vi "Read-Write Holding Registers.vi"(5 "write values":u16[](array[numeric]), 7 "write starting address":u16, 8 "error in (no error)":errorcluster, 9 "read quantity":u16, 10 "read starting address":u16, 11 "MB session in":refnum<class "MB_Master.lvclass">) -> (0 "error out":errorcluster, 2 "read registers":u16[](array[numeric]), 3 "MB session out":refnum<class "MB_Master.lvclass">)   [LabVIEW 2016, in "MB Master.lvlib"]
doc: "Function Code 23: Writes <b>write values</b> to holding registers starting at <b>write starting address</b> then reads <b>read quantity</b> number of holding registers starting at <b>read starting address</b>"
uses:
  MB Master.lvlib
  MB_Master.lvclass
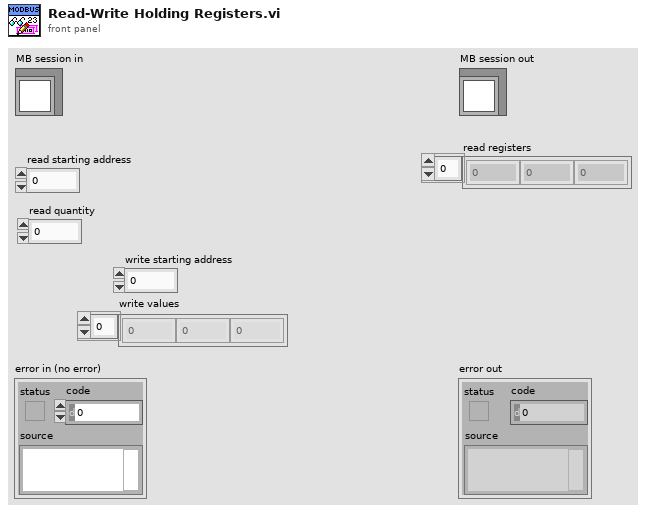
[diagram p1: front panel]
types:
  T1 = typedef "MB Master.lvlib/MB_PDU_Cluster.ctl" = cluster{"Function Code":u8, "Data":u8[], "RTU_DataBytes":i32}
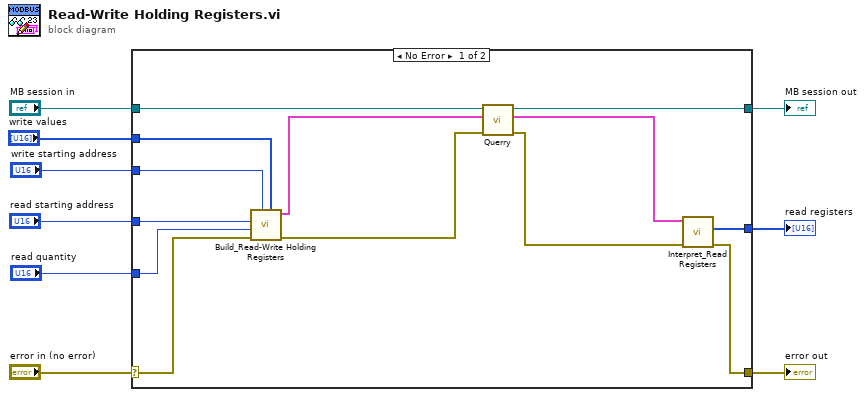
[diagram p0: block diagram]
diagram:
  n1 = case shown="No Error" "error in (no error)" {
    selector: "error in (no error)" -> [w14 w24]
    tunnel: [w21 w24] -> w8
    tunnel: [w19 w23] -> w6
    tunnel: "MB session in" -> [w18 w23]
    tunnel: "read starting address" -> [w16 _]
    tunnel: "read quantity" -> [w15 _]
    tunnel: [w20 _] -> w3
    tunnel: "write starting address" -> [w13 _]
    tunnel: "write values" -> [w12 _]
    frame No Error {
      n2 = call "Build_Read-Write Holding Registers.vi"("write values"=w12, "write starting address"=w13, "error in (no error)"=w14, "read quantity"=w15, "read starting address"=w16) -> ("error out"=w17:errorcluster, "MB_PDU"=w11:T1)  [unwired: 5 in]
      n3 = call-dynamic "Querry.vi"("error in (no error)"=w17, "PDU_req"=w11, "MB_Master in"=w18) -> ("error out"=w22:errorcluster, "PDU_resp"=w10:T1, "MB_Master out"=w19:refnum<class "MB_Master.lvclass">)  [unwired: 6 in]
      n4 = call "Interpret_Read Registers.vi"("error in (no error)"=w22, "MB_PDU_resp in"=w10) -> ("error out"=w21:errorcluster, "Registers"=w20:u16[])  [unwired: 8 in]
    }
    frame Error {
    }
  }
  "error out" <- w8
  "MB session out" <- w6
  "read registers" <- w3
